vi "Handling AI param_ext.vi"(4 "APCcode":i32[](array[numeric]), 5 "initialise":bool, 6 "AP":dbl[](array[numeric]), 7 "connect":bool[](array[boolean]), 8 "error in":errorcluster, 9 "input registers":u16[][](array[numeric]) format="%x", 10 "AI.AIP":refnum<data-value>, 11 "AI in":T1) -> (0 "error":errorcluster, 3 "AI out":T1)   [LabVIEW 2019, in "Inputs.lvlib"]
uses:
  Inputs.lvlib
  Ctl/AI short.ctl
  Ctl/Parameter State.ctl
  Sensor limits calc.vi
  Sensor 2P.vi
  Filter/Filter_ext.vi
  Trigers/RS32_ext.vi
  Param limits calc.vi
  Sensor_limit_Hd.vi
  Sensor_limit_Ld.vi
  Sensor_limit_H.vi
  Sensor_limit_L.vi
  Timer Delay/Timers.lvlib
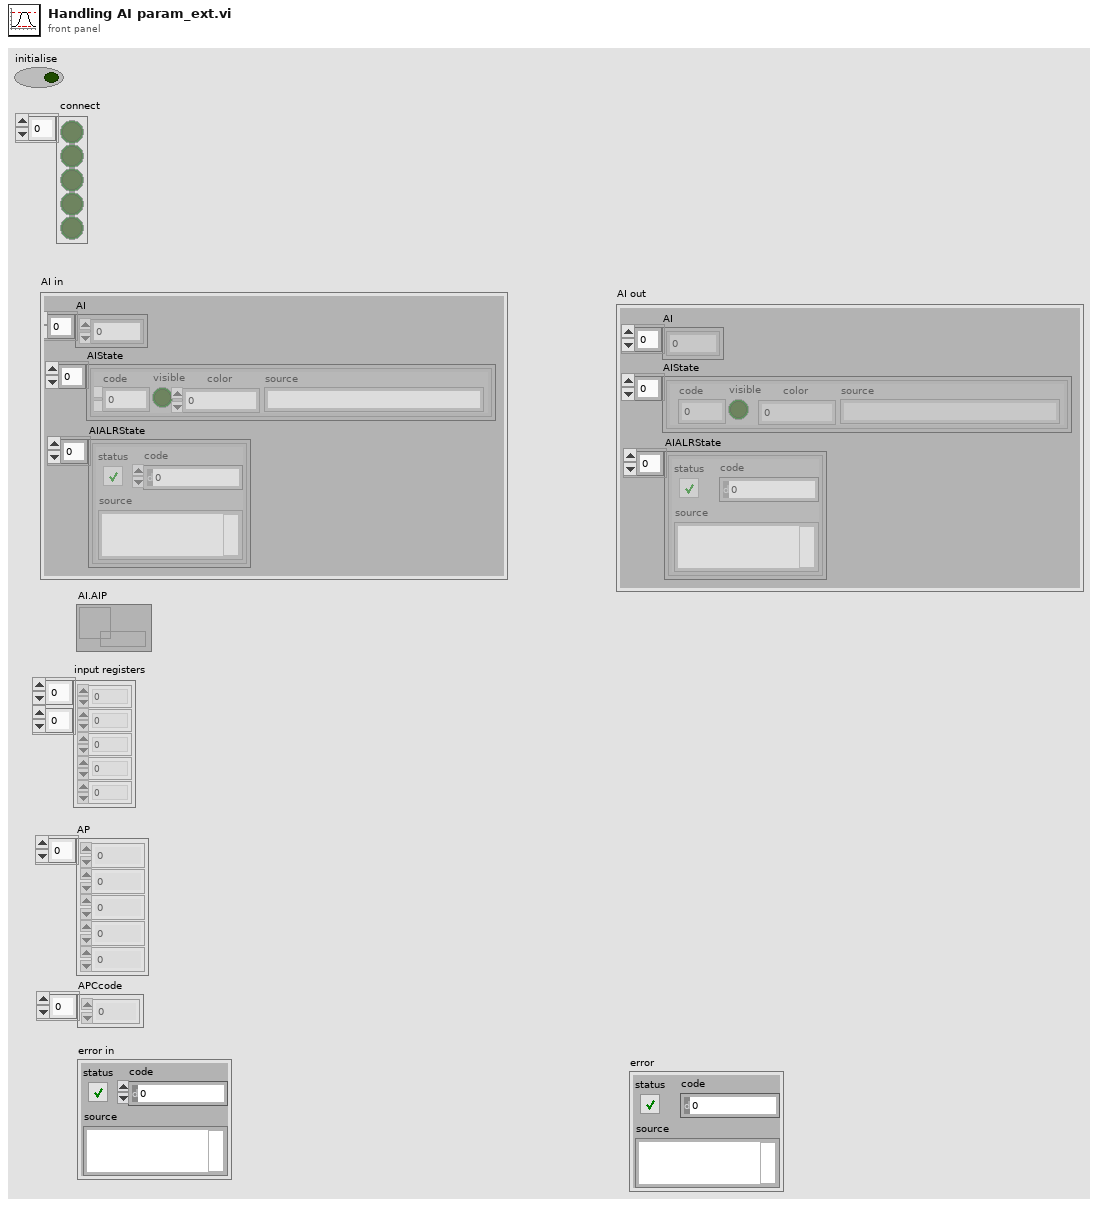
[diagram p1: front panel]
types:
  T1 = typedef "Inputs.lvlib/AI short.ctl" = cluster{"AI":dbl[], "AIState":T2[], "AIALRState":errorcluster[]}
  T2 = typedef "Inputs.lvlib/Parameter State.ctl" = cluster{"code":i32, "visible":bool, "color":u32, "source":string}
  T3 = cluster{"Filter PV_OUT":dbl, "Filter T":dbl, "Filter dT":dbl, "RS32 Q":u32}[]
  T4 = cluster{"Filter PV_OUT":dbl, "Filter T":dbl, "Filter dT":dbl, "RS32 Q":u32}
  T5 = cluster{"[0]":dbl, "[1]":dbl, "[2]":dbl, "[3]":dbl, "[4]":dbl, "[5]":dbl, "[6]":dbl, "[7]":dbl, "[8]":dbl, "[9]":dbl, "[10]":dbl, "[11]":dbl, "[12]":dbl, "[13]":dbl, "[14]":dbl, "[15]":dbl, "[16]":dbl, "[17]":dbl, "[18]":dbl, "[19]":dbl, "[20]":dbl}
  T6 = cluster{"[0]":dbl, "[1]":dbl, "[2]":dbl, "[3]":dbl, "[4]":dbl, "[5]":dbl, "[6]":dbl, "[7]":dbl, "[8]":dbl, "[9]":dbl, "[10]":dbl, "[11]":dbl, "[12]":dbl, "[13]":dbl, "[14]":dbl, "[15]":dbl, "[16]":dbl}
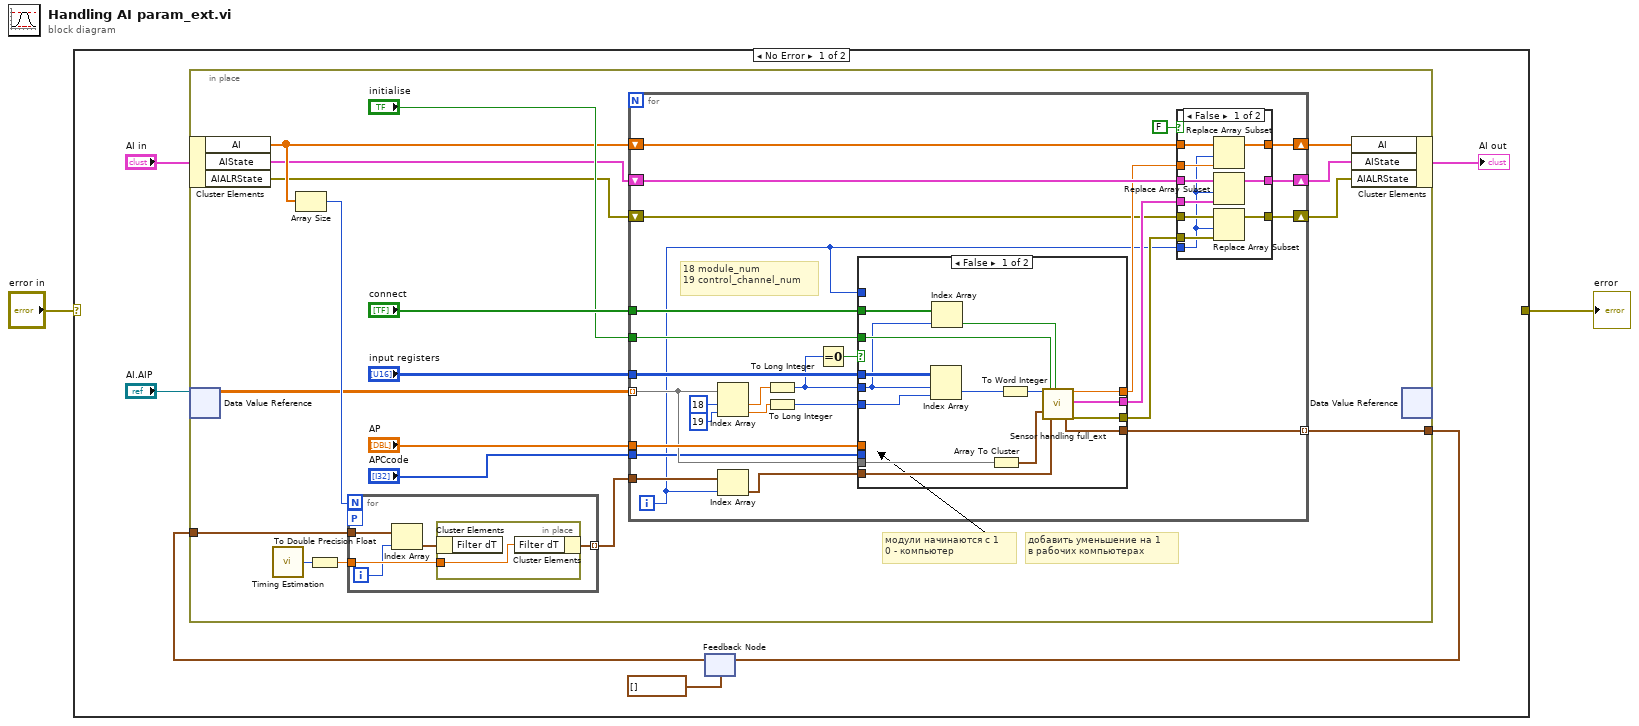
[diagram p0: block diagram]
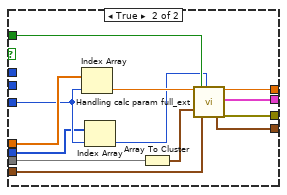
[diagram p2: hidden frame]
diagram:
  n1 = case shown="No Error" "error in" {
    selector: "error in" -> [_ w101]
    tunnel: [_ w101] -> w1
    frame No Error {
      n2 = feedback #1(T3 []) -> (w8:T3)
      n3 = in-place {
        in-place-border: w8 -> [w19]
        in-place-border: [w16] -> w6
        # "добавить уменьшение на 1\nв рабочих компьютерах"
        # "модули начинаются с 1\n0 - компьютер"
        n4 = in-place-cluster #2("AI in") -> ("AI"=w15:dbl[], "AIState"=w14:T2[], "AIALRState"=w13:errorcluster[])
        n5 = in-place-dvr #3("AI.AIP") -> (w12:dbl[][])  [unwired: 1 out]
        n6 = call "Timing Estimation.vi"() -> ("dt (ms) out"=w21:u32)  [unwired: 9 in]
        n7 = Array Size(array=w15) -> (size(s)=w17:i32)
        n8 = To Double Precision Float(number=w21) -> (double precision float=w20:dbl)
        n9 = for {
          N: w17 -> [_]
          tunnel: w20 -> [w30]
          workers-P: _ -> [_]
          tunnel: w19 -> [w29]
          tunnel: [w31] -> w18 mode=indexing
          i -> [w27]
          n10 = Index Array(array=w29, index=w27) -> (element=w28:T4)
          n11 = in-place {
            in-place-border: w30 -> [w32]
            n12 = in-place-cluster #4(w28) -> ()  [unwired: 1 out]
            n13 = in-place-cluster #4("Filter dT"=w32) -> (w31:T4)
          }
        }
        n14 = for {
          tunnel: w12 -> [w43] mode=indexing
          tunnel: "input registers" -> [w56]
          tunnel: "connect" -> [w52]
          shift-right: [w53] -> w11
          shift-left: w15 -> [w55]
          shift-right: [w58] -> w10
          shift-left: w14 -> [w59]
          shift-right: [w49] -> w9
          shift-left: w13 -> [w48]
          tunnel: "initialise" -> [w47]
          tunnel: "AP" -> [w44]
          tunnel: "APCcode" -> [w42]
          tunnel: [w36] -> w16 mode=indexing
          tunnel: w18 -> [w35]
          i -> [w33]
          # "18 module_num\n19 control_channel_num"
          n15 = Index Array(array=w43, index #1=18 ("index (col)"), index #2=19 ("index (col)")) -> (element #1=w38:dbl, element #2=w37:dbl)
          n16 = Index Array(array=w35, index=w33) -> (element=w34:T4)
          n17 = To Long Integer(number=w38) -> (32bit integer=w45:i32)
          n18 = To Long Integer(number=w37) -> (32bit integer=w41:i32)
          n19 = Equal To 0?(x=w45) -> (x = 0?=w46:bool)
          n20 = case shown="False" w46 {
            tunnel: w43 -> [w74 w86]
            tunnel: [w73 w83] -> w57
            tunnel: w56 -> [w72 _]
            tunnel: [w70 w84] -> w54
            tunnel: w52 -> [w69 _]
            tunnel: w45 -> [w64 _]
            tunnel: w41 -> [w67 w81]
            tunnel: w47 -> [w66 w82]
            tunnel: w33 -> [_ _]
            tunnel: w44 -> [_ w87]
            tunnel: w42 -> [_ w80]
            tunnel: [w65 w78] -> w40
            tunnel: w34 -> [w61 w76]
            tunnel: [w60 w75] -> w36
            frame False {
              n21 = Index Array(array=w72, index (row)=w64, index (col)=w67) -> (element=w71:u16)
              n22 = Index Array(array=w69, index=w64) -> (element=w68:bool)
              n23 = Array To Cluster(array=w74) -> (cluster=w62:T5)
              n24 = To Word Integer(number=w71) -> (16bit integer=w63:i16)
              n25 = call "Sensor handling full_ext.vi"("PV"=w63, "control"=w62, "initialise"=w66, "Sensor handling full reg old"=w61, "connect"=w68) -> ("Sensor handling full reg"=w60:T4, "PVOUT"=w70:dbl, "STATE"=w73:T2, "ALRSTATE"=w65:errorcluster)  [unwired: 9 in, 2 out]
            }
            frame True {
              n26 = Index Array(array=w87, index=w81) -> (element=w85:dbl)
              n27 = Index Array(array=w80, index=w81) -> (element=w79:i32)
              n28 = Array To Cluster(array=w86) -> (cluster=w77:T6)
              n29 = call "Handling calc param full_ext.vi"("PV"=w85, "control"=w77, "initialise"=w82, "Sensor handling full reg old"=w76, "code"=w79) -> ("Sensor handling full reg"=w75:T4, "PVOUT"=w84:dbl, "STATE"=w83:T2, "ALRSTATE"=w78:errorcluster)  [unwired: 9 in, 2 out]
            }
          }
          n30 = case shown="False" FALSE {
            tunnel: w59 -> [w97 w99]
            tunnel: [w96 w99] -> w58
            tunnel: w57 -> [w95 _]
            tunnel: w55 -> [w94 w100]
            tunnel: w54 -> [w92 _]
            tunnel: [w93 w100] -> w53
            tunnel: w33 -> [w88 _]
            tunnel: w40 -> [w91 _]
            tunnel: w48 -> [w90 w98]
            tunnel: [w89 w98] -> w49
            frame False {
              n31 = Replace Array Subset(array=w94, new element=w92, index=w88) -> (w93:dbl[])
              n32 = Replace Array Subset(array=w97, new element=w95, index=w88) -> (w96:T2[])
              n33 = Replace Array Subset(array=w90, new element=w91, index=w88) -> (w89:errorcluster[])
            }
            frame True {
            }
          }
        }
        n34 = in-place-cluster #2("AI"=w11, "AIState"=w10, "AIALRState"=w9) -> (→"AI out":T1)
        n35 = in-place-dvr #3() -> ()  [unwired: 1 in, 2 out]
      }
      n36 = feedback-in #1(w6) -> ()
    }
    frame Error {
    }
  }
  "error" <- w1
